vi "河内塔-绘图.vi"(0 "图片":picture, 5 "Value":u8[](array[numeric]), 7 "第几塔":i32, 9 "Width":u32, 11 "Height":u32, 13 "N":u8) -> (4 "新图片":picture)   [LabVIEW 2016]
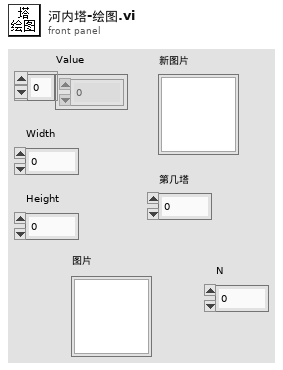
[diagram p1: front panel]
types:
  T1 = enum16{"User-specified Font", "Application Font", "System Font", "Dialog Font"}
  T2 = cluster{"Font Name:":string, "Size":i16, "Strikeout?":bool, "Italic?":bool, "Underline?":bool, "Outline?":bool, "Shadow?":bool, "Bold?":bool}
  T3 = cluster{"horizontal":enum16{"left", "center", "right"}, "vertical":enum16{"top", "center", "bottom"}}
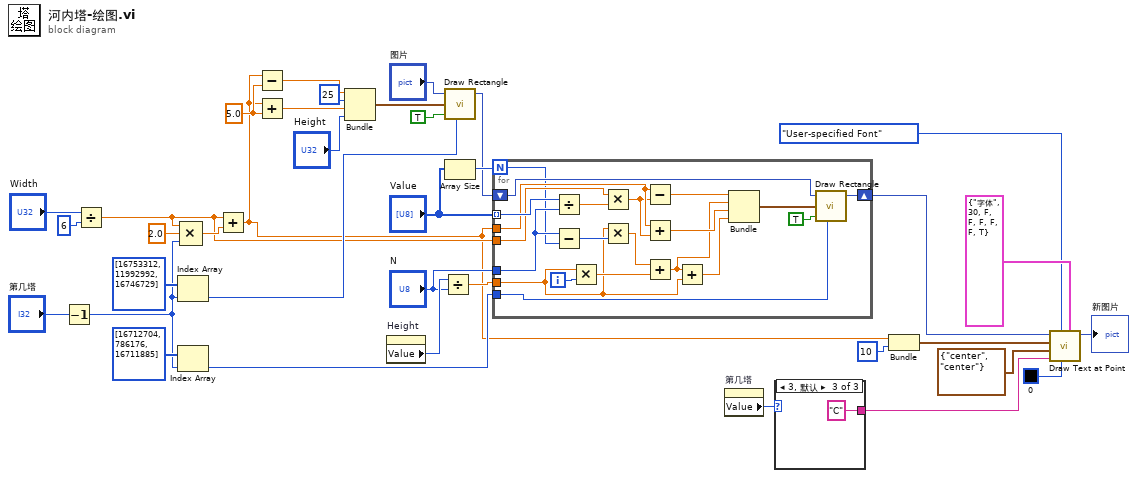
[diagram p0: block diagram]
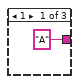
[diagram p2: hidden frame]
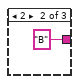
[diagram p3: hidden frame]
diagram:
  w36 = 5.0 ("y")
  n1 = Decrement(x="第几塔") -> (x-1=w19:i32)
  n2 = Divide(x="Width", y=u32 6) -> (x/y=w13:dbl)
  n3 = Index Array(array=u32[] [16753312, 11992992, 16746729], index=w19) -> (element=w21:u32)
  n4 = Index Array(array=u32[] [16712704, 786176, 16711885], index=w19) -> (element=w18:u32)
  n5 = Compound Arithmetic op=MULTIPLY(w13, 2.0 ("值"), w19) -> (w17:dbl)
  n6 = Add(x=w13, y=w17) -> (x+y=w6:dbl)
  n7 = Subtract(x=w6, y=w36) -> (x-y=w33:dbl)
  n8 = Add(x=w6, y=w36) -> (x+y=w35:dbl)
  n9 = Bundle(w33, 25, w35, "Height"="Height") -> (w29:cluster{dbl, i32, dbl, "Height":u32})  [unwired: 1 in]
  n10 = property on="Height" class="DigNum (严格)"() -> ("Value"=w16:u32)  [unwired: 2 in, 2 out]
  n11 = Divide(x=w16, y="N") -> (x/y=w14:dbl)
  n12 = call <vilib>:"Draw Rectangle.vi"("picture"="图片", "rect"=w29, "fill?(F)"=TRUE, "color(black)"=w21) -> ("new picture"=w23:picture)  [unwired: 5 in]
  n13 = Array Size(array="Value") -> (size(s)=w26:i32)
  n14 = for {
    N: w26 -> [w39]
    tunnel: "Value" -> [w55] mode=indexing
    shift-right: [w37] -> w12
    shift-left: w23 -> [w56]
    tunnel: w18 -> [w57]
    tunnel: w13 -> [w53]
    tunnel: w6 -> [w51]
    tunnel: "N" -> [w48]
    tunnel: w14 -> [w41]
    i -> [w38]
    n15 = Divide(x=w55, y=w48) -> (x/y=w54:dbl)
    n16 = Subtract(x=w48, y=w39) -> (x-y=w47:i32)
    n17 = Multiply(x=w41, y=w38) -> (x*y=w44:dbl)
    n18 = Multiply(x=w53, y=w54) -> (x*y=w50:dbl)
    n19 = Multiply(x=w41, y=w47) -> (x*y=w45:dbl)
    n20 = Subtract(x=w51, y=w50) -> (x-y=w52:dbl)
    n21 = Add(x=w51, y=w50) -> (x+y=w49:dbl)
    n22 = Add(x=w45, y=w44) -> (x+y=w42:dbl)
    n23 = Add(x=w42, y=w41) -> (x+y=w43:dbl)
    n24 = Bundle(w52, w42, w49, w43) -> (w46:cluster{dbl, dbl, dbl, dbl})  [unwired: 1 in]
    n25 = call <vilib>:"Draw Rectangle.vi"("picture"=w56, "rect"=w46, "fill?(F)"=TRUE, "color(black)"=w57) -> ("new picture"=w37:picture)  [unwired: 5 in]
  }
  n26 = property on="第几塔" class="DigNum (严格)"() -> ("Value"=w3:i32)  [unwired: 2 in, 2 out]
  n27 = case shown="3, 默认" w3 {
    tunnel: ["A" "B" "C"] -> w8
    frame 1 {
    }
    frame 2 {
    }
    frame 3, Default {
    }
  }
  n28 = Bundle(w6, 10) -> (w10:cluster{dbl, i32})  [unwired: 1 in]
  n29 = call <vilib>:"Draw Text at Point.vi"("[user-specified font]"=T2 {"Font Name:"="字体", "Size"=30, "Strikeout?"=FALSE, "Italic?"=FALSE, "Underline?"=FALSE, "Outline?"=FALSE, "Shadow?"=FALSE, "Bold?"=TRUE}, "text color(black)"=u32 0, "desired font(Application)"=T1."User-specified Font", "text"=w8, "alignment(left, top)"=T3 {"horizontal"=enum."center", "vertical"=enum."center"}, "origin"=w10, "picture"=w12) -> ("new picture"=→"新图片":picture)  [unwired: 3 in, 1 out]
